vi "Get SMO RC Type.vi"(8 "error in (no error)":errorcluster, 11 "ExampleInstrument in":refnum<class "Instrument.Framework-Template.lvclass">) -> (0 "error out":errorcluster, 2 "Dependencies.RemoteControl":refnum<class "RemoteControl.lvclass">, 3 "ExampleInstrument out":refnum<class "Instrument.Framework-Template.lvclass">)   [LabVIEW 2019, in "Instrument.Framework-Template.lvclass"]
uses:
  Instrument.Framework-Template.lvclass
  <userlib>/LevyLab/RemoteControl/RemoteControl.lvclass
  Framework/Instrument Types/SCPI/Instrument.SCPI.lvclass
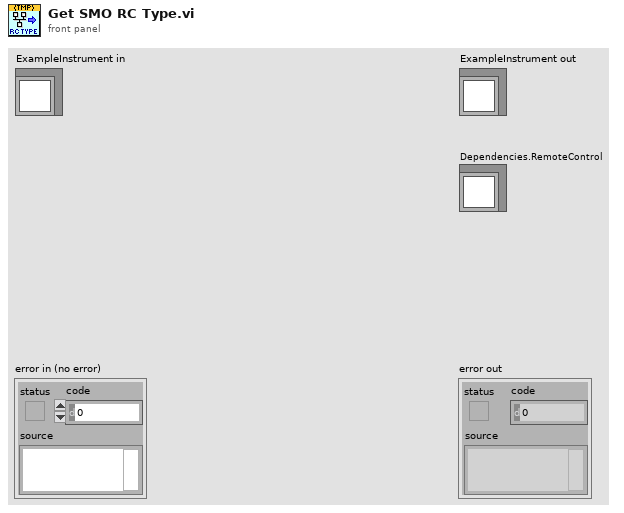
[diagram p1: front panel]
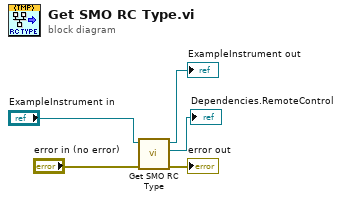
[diagram p0: block diagram]
diagram:
  n1 = call-parent "Get SMO RC Type.vi"("error in (no error)"="error in (no error)", "Instrument in"="ExampleInstrument in") -> ("error out"=→"error out":errorcluster, "RemoteControl.lvclass"=→"Dependencies.RemoteControl":refnum<class "RemoteControl.lvclass">, "Instrument out"=→"ExampleInstrument out":refnum<class "Instrument.Framework-Template.lvclass">)  [unwired: 7 in]
